vi "Wfm Converter.vi"(8 "Select":u8, 9 "Sample In":fxp<+/-,8,8>) -> (1 "Sample Out":fxp<+/-,8,8>)   [LabVIEW 2015]
doc: "Modifies the shape of the input sine wave, allowing to select between 4 different output waveforms:\n' 0 ' _______ Sine (untouched)\n' 1 ' _______ Square\n' 2 ' _______ Triangle\n' 3 ' _______ Sawtooth"
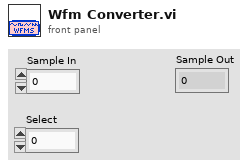
[diagram p1: front panel]
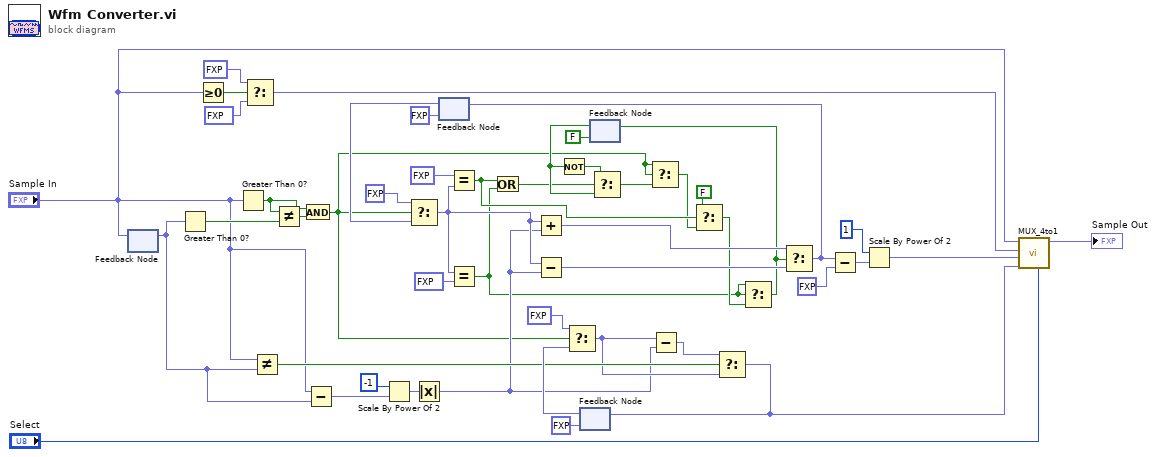
[diagram p0: block diagram]
diagram:
  n1 = feedback #1() -> (w36:fxp<+/-,8,8>)  [unwired: 1 in]
  n2 = feedback-in #1("Sample In") -> ()
  n3 = Greater Than 0?(x=w36) -> (x > 0?=w40:bool)
  n4 = Greater Or Equal To 0?(x="Sample In") -> (x >= 0?=w45:bool)
  n5 = Greater Than 0?(x="Sample In") -> (x > 0?=w42:bool)
  n6 = Select(t=fxp<+/-,8,8> 124.0 ("m_axis_data_tdata"), s=w45, f=fxp<+/-,8,8> -125.0 ("m_axis_data_tdata")) -> (s? t:f=w6:fxp<+/-,8,8>)
  n7 = Not Equal?(x="Sample In", y=w36) -> (x != y?=w38:bool)
  n8 = Not Equal?(x=w42, y=w40) -> (x != y?=w41:bool)
  n9 = And(x=w42, y=w41) -> (x .and. y?=w17:bool)
  n10 = Subtract(x="Sample In", y=w36) -> (x-y=w33:fxp<+/-,8,8>)
  n11 = Scale By Power Of 2(n=i16 -1, x=w33) -> (x*2^n=w32:fxp<+/-,8,8>)
  n12 = Absolute Value(x=w32) -> (abs(x)=w20:fxp<+,8,8>)
  n13 = feedback #2(fxp<+/-,8,8> 0.0) -> (w30:fxp<+/-,8,8>)
  n14 = Select(t=fxp<+/-,8,8> 0.0, s=w17, f=w30) -> (s? t:f=w21:fxp<+/-,8,8>)
  n15 = Equal?(x=fxp<+/-,8,8> 127.0, y=w21) -> (x = y?=w15:bool)
  n16 = Equal?(x=w21, y=fxp<+/-,8,8> -128.0) -> (x = y?=w1:bool)
  n17 = Or(x=w15, y=w1) -> (x .or. y?=w23:bool)
  n18 = Add(x=w21, y=w20) -> (x+y=w19:fxp<+/-,8,8>)
  n19 = Subtract(x=w21, y=w20) -> (x-y=w22:fxp<+/-,8,8>)
  n20 = feedback #3(fxp<+/-,8,8> -1.0) -> (w44:fxp<+/-,8,8>)
  n21 = Select(t=fxp<+/-,8,8> 127.0 ("m_axis_data_tdata"), s=w17, f=w44) -> (s? t:f=w35:fxp<+/-,8,8>)
  n22 = feedback #4(FALSE) -> (w26:bool)
  n23 = Not(x=w26) -> (.not. x?=w27:bool)
  n24 = Select(t=w27, s=w23, f=w26) -> (s? t:f=w16:bool)
  n25 = Select(t=w17, s=w17, f=w16) -> (s? t:f=w13:bool)
  n26 = Subtract(x=w35, y=w20) -> (x-y=w34:fxp<+/-,8,8>)
  n27 = Select(t=FALSE ("x = y?"), s=w15, f=w13) -> (s? t:f=w12:bool)
  n28 = Select(t=w34, s=w38, f=w35) -> (s? t:f=w4:fxp<+/-,8,8>)
  n29 = feedback-in #3(w4) -> ()
  n30 = Select(t=w1, s=w1, f=w12) -> (s? t:f=w11:bool)
  n31 = feedback-in #4(w11) -> ()
  n32 = Select(t=w19, s=w11, f=w22) -> (s? t:f=w10:fxp<+/-,8,8>)
  n33 = feedback-in #2(w10) -> ()
  n34 = Subtract(x=w10, y=fxp<+/-,8,8> 64.0) -> (x-y=w8:fxp<+/-,8,8>)
  n35 = Scale By Power Of 2(n=i16 1, x=w8) -> (x*2^n=w5:fxp<+/-,8,8>)
  n36 = call "MUX_4to1.vi"("Select"="Select", "Input 3"=w4, "Input 2"=w5, "Input 1"=w6, "Input 0"="Sample In") -> ("Output"=→"Sample Out":fxp<+/-,8,8>)  [unwired: 6 in]
